vi "micro.vi"() -> ()   [LabVIEW 2015]
uses:
  <vilib>/Platform/TimedLoop/XDataNode/timing_clust.ctl
  <vilib>/Platform/TimedLoop/XDataNode/nitl_modes.ctl
  <vilib>/Platform/TimedLoop/XDataNode/wakeup.ctl
  <vilib>/Platform/TimedLoop/XDataNode/XDataNode.xnode
  <vilib>/Platform/TimedLoop/XDataNode/XDNodeRunTimeDep.lvlib
panel:
  out ":":dbl
  out "?":dbl format="%_4f"
  out ":":dbl
  out ":":dbl
  out "?":bool
  # "CRONOMETRO"
  # "SET"
  # "TIME"
  # "RESET"
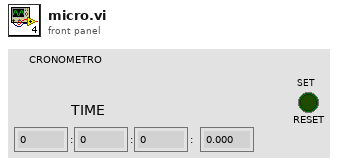
[diagram p1: front panel]
types:
  T1 = typedef "XDNodeRunTimeDep.lvlib/timing_clust.ctl" = cluster{"Expected End [f-1]":u64, "Actual End [f-1]":u64, "Finished Late? [f-1]":bool, "Expected End [i-1]":u64, "Actual End [i-1]":u64, "Finished Late? [i-1]":bool, "Expected Start [i]":u64, "Actual Start [i]":u64, "Expected Start [f]":u64, "Actual Start [f]":u64, "Source Name":string, "Structure Name":string, "Period":i64, "Deadline":i64, "Offset":i64, "Start":i64, "Priority":i32, "Timeout":i32, "Mode":T2, "Wakeup Reason":T3, "Error":errorcluster, "Source Type":string, "Secondary Source Type":string, "Global End Time":u64, "Global Start Time":u64, "Frame Duration":u64, "Iteration Duration":u64, "Assigned CPU":i32, "I/O Scan Engine Mode":u32}
  T2 = typedef "XDNodeRunTimeDep.lvlib/nitl_modes.ctl" = enum32{"No Change", "Process missed periods, maintain original phase", "Discard missed periods, maintain original phase", "Process missed periods, ignore original phase", "Discard missed periods, ignore original phase"}
  T3 = typedef "XDNodeRunTimeDep.lvlib/wakeup.ctl" = enum32{"Normal", "Aborted", "Asynchronous wakeup", "Timing source error", "Timed loop error", "Timeout"}
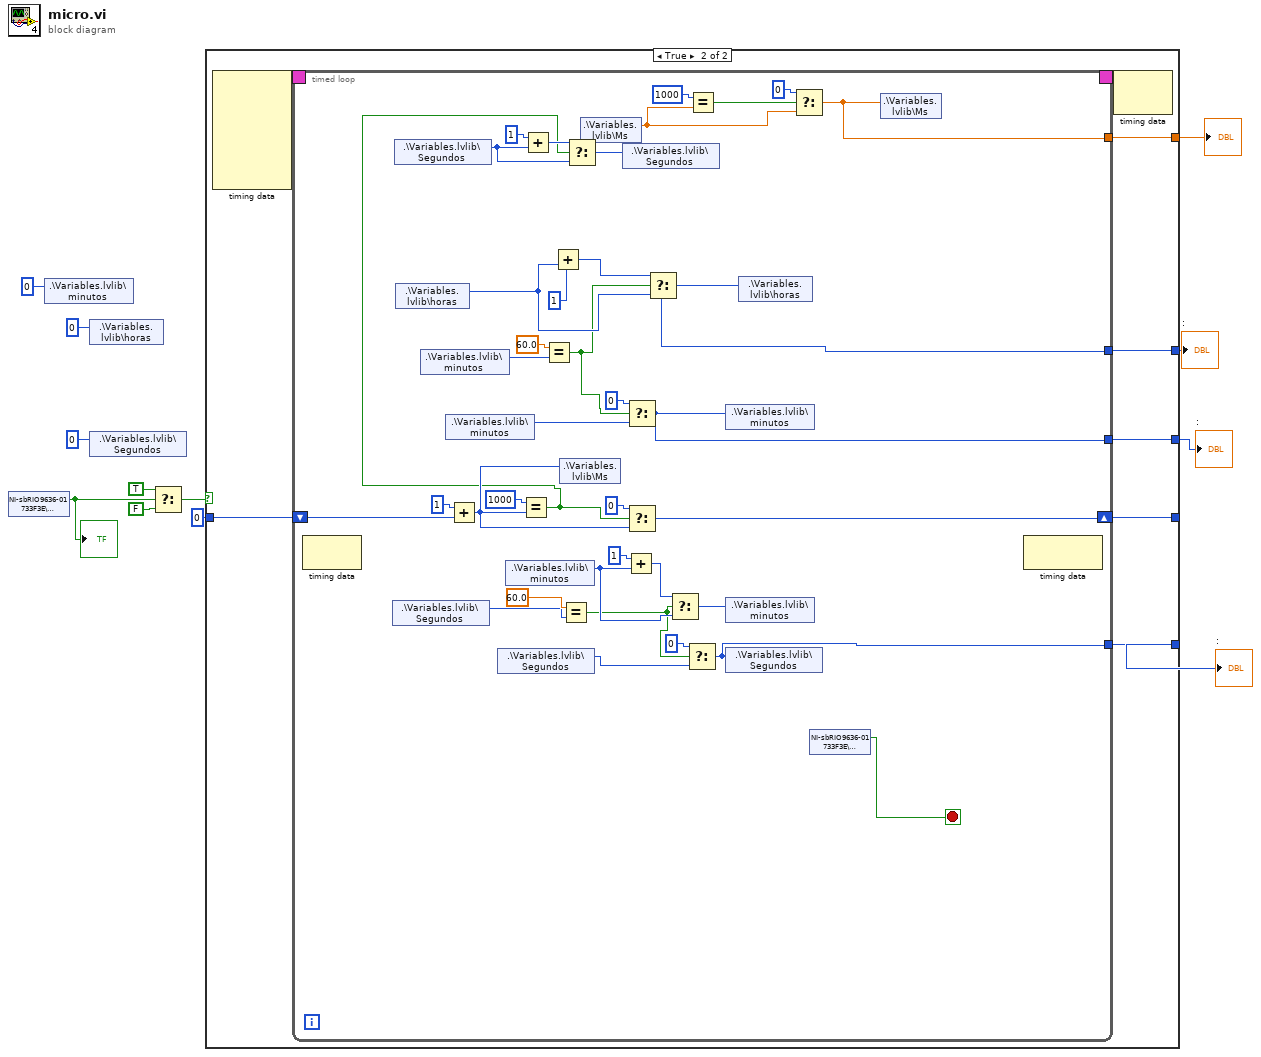
[diagram p0: block diagram]
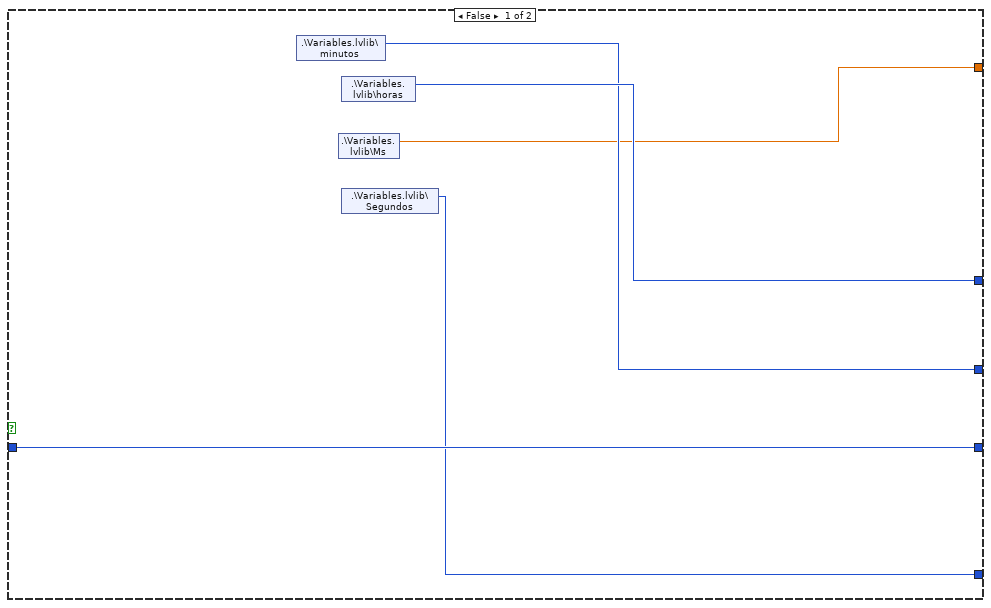
[diagram p2: hidden frame]
diagram:
  n1 = shared-variable "NI-sbRIO9636-01733F3E\\User-Defined Variables\\Set"() -> (w5:bool)  [unwired: 1 in, 1 out]
  "?" <- w5
  n2 = shared-variable ".\\Variables.lvlib\\minutos"(i16 0 ("minutos")) -> ()  [unwired: 1 in, 1 out]
  n3 = shared-variable ".\\Variables.lvlib\\horas"(i16 0 ("horas")) -> ()  [unwired: 1 in, 1 out]
  n4 = shared-variable ".\\Variables.lvlib\\Segundos"(i16 0 ("Segundos")) -> ()  [unwired: 1 in, 1 out]
  n5 = Select(t=TRUE, s=w5, f=FALSE) -> (s? t:f=w6:bool)
  n6 = case shown="True" w6 {
    tunnel: 0 -> [w17 w22]
    tunnel: [w17 w23] -> _
    tunnel: [w16 w21] -> w4
    tunnel: [w14 w20] -> w3
    tunnel: [w15 w19] -> w2
    tunnel: [w13 w18] -> w1
    frame False {
      n7 = shared-variable ".\\Variables.lvlib\\minutos"() -> (w14:i16)  [unwired: 1 in, 1 out]
      n8 = shared-variable ".\\Variables.lvlib\\Ms"() -> (w13:dbl)  [unwired: 1 in, 1 out]
      n9 = shared-variable ".\\Variables.lvlib\\horas"() -> (w15:i16)  [unwired: 1 in, 1 out]
      n10 = shared-variable ".\\Variables.lvlib\\Segundos"() -> (w16:i16)  [unwired: 1 in, 1 out]
    }
    frame True {
      n11 = node-c288() -> (w25:T1)  [unwired: 6 in]
      n12 = timed-loop {
        timing: w25 -> [_]
        timing-out: [_] -> w24
        shift-right: [w35] -> w23
        shift-left: w22 -> [w38]
        tunnel: [w29] -> w21
        tunnel: [w28] -> w20
        tunnel: [w27] -> w19
        tunnel: [w26] -> w18
        stop <- w61 stop-if-true
        n13 = node-c288() -> ()  [unwired: 1 in, 1 out]
        n14 = shared-variable ".\\Variables.lvlib\\Segundos"() -> (w57:i16)  [unwired: 1 in, 1 out]
        n15 = shared-variable ".\\Variables.lvlib\\Segundos"() -> (w50:i16)  [unwired: 1 in, 1 out]
        n16 = shared-variable ".\\Variables.lvlib\\horas"() -> (w48:i16)  [unwired: 1 in, 1 out]
        n17 = shared-variable ".\\Variables.lvlib\\minutos"() -> (w53:i16)  [unwired: 1 in, 1 out]
        n18 = shared-variable ".\\Variables.lvlib\\minutos"() -> (w46:i16)  [unwired: 1 in, 1 out]
        n19 = Add(x=1, y=w38) -> (x+y=w34:i32)
        n20 = shared-variable ".\\Variables.lvlib\\Segundos"() -> (w44:i16)  [unwired: 1 in, 1 out]
        n21 = shared-variable ".\\Variables.lvlib\\minutos"() -> (w49:i16)  [unwired: 1 in, 1 out]
        n22 = Equal?(x=i16 1000, y=w34) -> (x = y?=w30:bool)
        n23 = Add(x=1, y=w50) -> (x+y=w59:i32)
        n24 = Equal?(x=60.0, y=w53) -> (x = y?=w32:bool)
        n25 = Add(x=1, y=w48) -> (x+y=w51:i32)
        n26 = shared-variable ".\\Variables.lvlib\\Ms"(w34) -> ()  [unwired: 1 in, 1 out]
        n27 = Equal?(x=60.0, y=w57) -> (x = y?=w31:bool)
        n28 = Select(t=w59, s=w30, f=w50) -> (s? t:f=w39:i32)
        n29 = shared-variable ".\\Variables.lvlib\\Ms"() -> (w40:dbl)  [unwired: 1 in, 1 out]
        n30 = shared-variable ".\\Variables.lvlib\\Segundos"(w39) -> ()  [unwired: 1 in, 1 out]
        n31 = Add(x=1, y=w49) -> (x+y=w55:i32)
        n32 = Select(t=0, s=w32, f=w46) -> (s? t:f=w28:i32)
        n33 = Select(t=0, s=w30, f=w34) -> (s? t:f=w35:i32)
        n34 = Select(t=w51, s=w32, f=w48) -> (s? t:f=w27:i32)
        n35 = Select(t=w55, s=w31, f=w49) -> (s? t:f=w33:i32)
        n36 = Select(t=0, s=w31, f=w44) -> (s? t:f=w29:i32)
        n37 = Equal?(x=i16 1000, y=w40) -> (x = y?=w41:bool)
        n38 = shared-variable ".\\Variables.lvlib\\minutos"(w28) -> ()  [unwired: 1 in, 1 out]
        n39 = shared-variable ".\\Variables.lvlib\\minutos"(w33) -> ()  [unwired: 1 in, 1 out]
        n40 = shared-variable ".\\Variables.lvlib\\Segundos"(w29) -> ()  [unwired: 1 in, 1 out]
        n41 = shared-variable ".\\Variables.lvlib\\horas"(w27) -> ()  [unwired: 1 in, 1 out]
        n42 = Select(t=0, s=w41, f=w40) -> (s? t:f=w26:dbl)
        n43 = shared-variable "NI-sbRIO9636-01733F3E\\User-Defined Variables\\On"() -> (w61:bool)  [unwired: 1 in, 1 out]
        n44 = shared-variable ".\\Variables.lvlib\\Ms"(w26) -> ()  [unwired: 1 in, 1 out]
        n45 = node-c288() -> ()  [unwired: 1 in, 1 out]
      }
      n46 = node-c288(w24) -> ()  [unwired: 1 out]
    }
  }
  ":" <- w4
  ":" <- w3
  ":" <- w2
  "?" <- w1
